vi "VISA Factory.vi"(8 "error in (no error)":errorcluster, 10 "settings":T1) -> (0 "error out":errorcluster, 3 "protocol out":refnum<class "Protocol Parent.lvclass">)   [LabVIEW 2019, in "Instrument Addon Scripting API.lvlib"]
doc: "Instantiates a new VISA Protocol object using the provided VISA settings."
uses:
  Instrument Addon Scripting API.lvlib
  Addon/Support Libraries/Protocols.lvlibp/Protocol Parent/Protocol Parent.lvclass
  Addon/Support Libraries/Protocols.lvlibp/VISA/VISA Settings.ctl
  Addon/Support Libraries/Protocols.lvlibp/VISA/VISA.lvclass
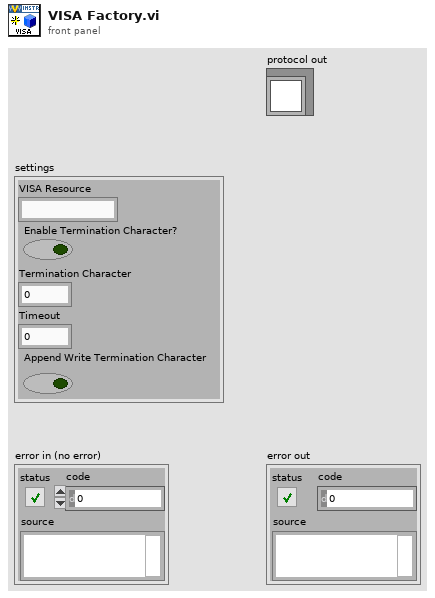
[diagram p1: front panel]
types:
  T1 = typedef "Protocols.lvlibp/VISA.lvclass/VISA Settings.ctl" = cluster{"VISA Resource":string, "Enable Termination Character?":bool, "Termination Character":u8, "Timeout":u32, "Append Write Termination Character":bool}
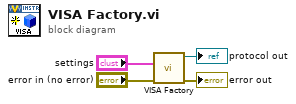
[diagram p0: block diagram]
diagram:
  n1 = call "VISA Factory.vi"("error in (no error)"="error in (no error)", "VISA settings"="settings") -> ("error out"=→"error out":errorcluster, "protocol out"=→"protocol out":refnum<class "Protocol Parent.lvclass">)  [unwired: 8 in]
